vi "Send Message.vi"(6 "timeout in ms (-1)":i32=-1, 8 "error in (no error)":errorcluster, 9 "Message in":refnum<class "Abstract Message.lvclass">, 10 "Consumer in":string, 11 "Abstract Producer in":refnum<class "Abstract Producer.lvclass">) -> (0 "error out":errorcluster, 1 "Message out":refnum<class "Abstract Message.lvclass">, 3 "Abstract Producer out":refnum<class "Abstract Producer.lvclass">, 4 "timed out?":bool)   [LabVIEW 2027, in "Messaging.lvlib" / "Abstract Producer.lvclass"]
uses:
  Abstract Producer.lvclass
  Message/Abstract Message/Abstract Message.lvclass
  Abstract Producer.lvclass/Abstract Producer.ctl
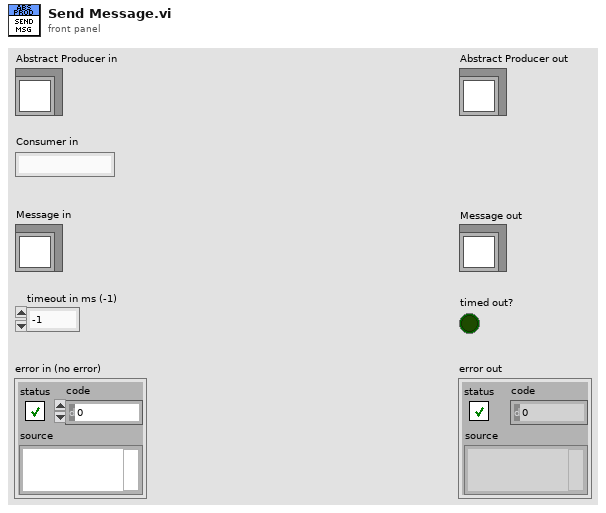
[diagram p1: front panel]
types:
  T1 = typedef "Messaging.lvlib/Abstract Producer.lvclass/Consumer Information.ctl" = cluster{"Name":string, "Request Queue":refnum<class "Abstract Message Queue.lvclass">, "Response Queue":refnum<class "Abstract Message Queue.lvclass">}
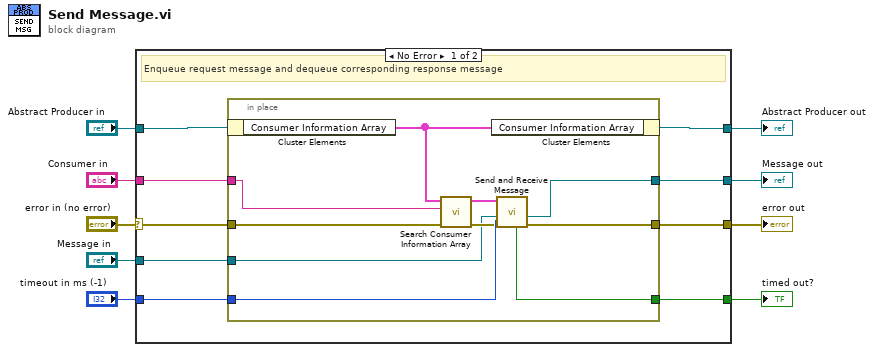
[diagram p0: block diagram]
diagram:
  n1 = case shown="No Error" "error in (no error)" {
    selector: "error in (no error)" -> [w14 w30]
    tunnel: [w13 w30] -> w8
    tunnel: [w17 w29] -> w6
    tunnel: "Abstract Producer in" -> [w18 w29]
    tunnel: "Consumer in" -> [w16 _]
    tunnel: "Message in" -> [w15 _]
    tunnel: [w12 _] -> w3
    tunnel: "timeout in ms (-1)" -> [w11 _]
    tunnel: [w10 _] -> w1
    frame No Error {
      # "Enqueue request message and dequeue corresponding response message"
      n2 = in-place {
        in-place-border: w16 -> [w28]
        in-place-border: w15 -> [w19]
        in-place-border: w14 -> [w26]
        in-place-border: [w21] -> w13
        in-place-border: [w20] -> w12
        in-place-border: w11 -> [w24]
        in-place-border: [w23] -> w10
        n3 = in-place-cluster #1(w18) -> ("Consumer Information Array"=w27:T1[])
        n4 = call "Search Consumer Information Array.vi"("error in (no error)"=w26, "Consumer in"=w28, "Consumer Information Array in"=w27) -> ("error out"=w22:errorcluster, "Consumer Information out"=w25:T1)  [unwired: 7 in]
        n5 = in-place-cluster #1("Consumer Information Array"=w27) -> (w17:refnum<class "Abstract Producer.lvclass">)
        n6 = call "Send and Receive Message.vi"("timeout in ms (-1)"=w24, "error in"=w22, "Message in"=w19, "Consumer Information"=w25) -> ("error out"=w21:errorcluster, "Message out"=w20:refnum<class "Abstract Message.lvclass">, "timed out?"=w23:bool)  [unwired: 5 in]
      }
    }
    frame Error {
    }
  }
  "error out" <- w8
  "Abstract Producer out" <- w6
  "Message out" <- w3
  "timed out?" <- w1
